vi "Model - Get States.vi"(8 "error in (no error)":errorcluster, 11 "View Model":T2) -> (0 "error out":errorcluster, 1 "CarWash Next State":T1, 2 "CarWash State":T1, 3 "View Model":T2)   [LabVIEW 2017]
doc: "Get Car wash states from DVR"
uses:
  Controls/View Model.ctl
  Configuration Database/Controls/Config Model.ctl
  Configuration Database/Controls/Congif Data.ctl
  Configuration Database/Controls/Config Commands.ctl
  Controls/Shared Model.ctl
  Error Handler/Controls/Error Model.ctl
  Error Handler/Controls/Error Data.ctl
  Error Handler/Controls/Error Type.ctl
  Car Wash Controller/Controls/Car Wash Model.ctl
  Car Wash Controller/Controls/Car Wash States.ctl
  Car Wash Controller/Controls/Controller Overhead.ctl
  Car Wash Controller/Controls/Vehicle Location.ctl
  Car Wash Controller/Controls/CarWash CMD.ctl
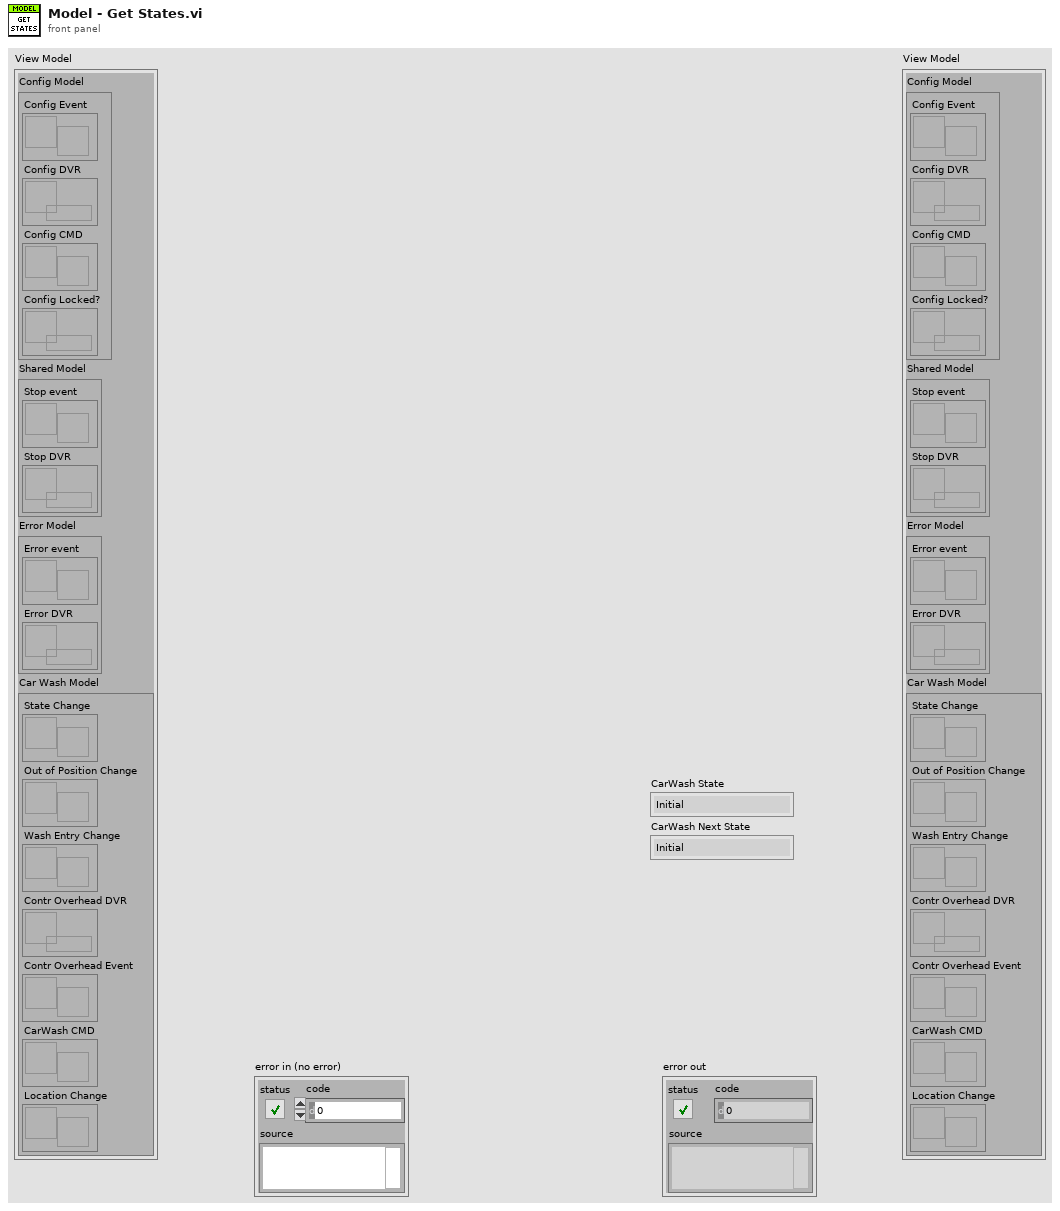
[diagram p1: front panel]
types:
  T1 = typedef "Car Wash States.ctl" = enum16{"Initial", "Wait for start", "Start", "Wait for vehicle", "Wash Step Execution", "Wash Step Complete", "Wash Cycle Complete", "Wash Exit", "Wash Abort", "Terminate"}
  T2 = typedef "View Model.ctl" = cluster{"Config Model":T3, "Shared Model":T4, "Error Model":T5, "Car Wash Model":T6}
  T3 = typedef "Config Model.ctl" = cluster{"Config Event":refnum<user-event>, "Config DVR":refnum<data-value>, "Config CMD":refnum<user-event>, "Config Locked?":refnum<data-value>}
  T4 = typedef "Shared Model.ctl" = cluster{"Stop event":refnum<user-event>, "Stop DVR":refnum<data-value>}
  T5 = typedef "Error Model.ctl" = cluster{"Error event":refnum<user-event>, "Error DVR":refnum<data-value>}
  T6 = typedef "Car Wash Model.ctl" = cluster{"State Change":refnum<user-event>, "Out of Position Change":refnum<user-event>, "Wash Entry Change":refnum<user-event>, "Contr Overhead DVR":refnum<data-value>, "Contr Overhead Event":refnum<user-event>, "CarWash CMD":refnum<user-event>, "Location Change":refnum<user-event>}
  T7 = typedef "Controller Overhead.ctl" = cluster{"State change":bool, "Location change":bool, "Vehicle out change":bool, "Wash entry change":bool, "Vehicle Location":T8, "CarWash State":T1, "CarWash Next State":T1}
  T8 = typedef "Vehicle Location.ctl" = enum16{"Entry", "Station 1", "Station 2", "Station 3", "Exit"}
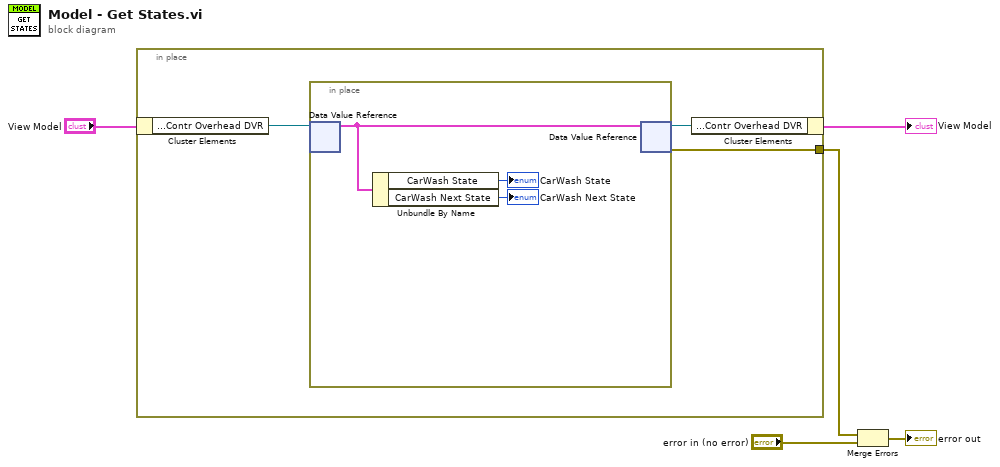
[diagram p0: block diagram]
diagram:
  n1 = in-place {
    in-place-border: [w6] -> w3
    n2 = in-place-cluster #1("View Model") -> ("Car Wash Model.Contr Overhead DVR"=w8:refnum<data-value>)
    n3 = in-place {
      n4 = in-place-dvr #2(w8) -> (w11:T7)  [unwired: 1 out]
      n5 = Unbundle By Name(w11) -> ("CarWash State"=→"CarWash State":T1, "CarWash Next State"=→"CarWash Next State":T1)
      n6 = in-place-dvr #2(w11) -> (w7:refnum<data-value>, w6:errorcluster)
    }
    n7 = in-place-cluster #1("Car Wash Model.Contr Overhead DVR"=w7) -> (→"View Model":T2)
  }
  n8 = Merge Errors(w3, "error in (no error)") -> (→"error out":errorcluster)
